vi "stripElementTags.vi"(8 "error in (no error)":errorcluster, 10 "XMLContents In":string, 11 "ReadElement in":refnum<class "XMLParser.lvclass">) -> (0 "error out":errorcluster, 1 "Contents":string, 2 "ParentTag":string, 3 "ReadElement out":refnum<class "XMLParser.lvclass">)   [LabVIEW 2014, in "XML.lvlib" / "XMLParser.lvclass"]
doc: "This method checks the open and close tags, and returns whatever is in the middle. This will not work if there are attributes in the parent tag."
uses:
  <userlib>/Common/XML/XMLParser/XMLParser.lvclass
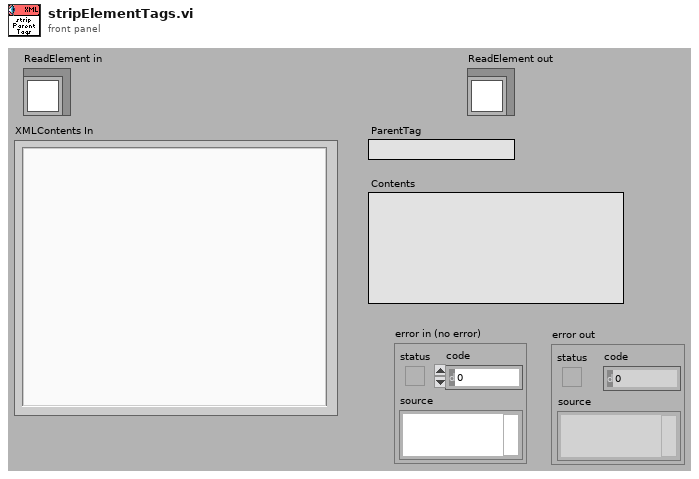
[diagram p1: front panel]
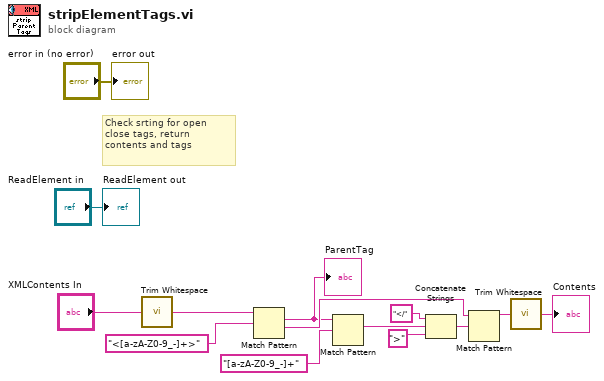
[diagram p0: block diagram]
diagram:
  # "Check srting for open close tags, return contents and tags"
  n1 = call <vilib>:"Trim Whitespace.vi"("string"="XMLContents In") -> ("trimmed string"=w11:string)  [unwired: 1 in]
  n2 = Match Pattern(string=w11, regular expression="<[a-zA-Z0-9_-]+>") -> (match substring=w5:string, after substring=w10:string)  [unwired: 1 in, 2 out]
  "ParentTag" <- w5
  n3 = Match Pattern(string=w5, regular expression="[a-zA-Z0-9_-]+") -> (match substring=w7:string)  [unwired: 1 in, 3 out]
  n4 = Concatenate Strings("</" ("string"), w7, ">" ("string")) -> (w8:string)
  n5 = Match Pattern(string=w10, regular expression=w8) -> (before substring=w12:string)  [unwired: 1 in, 3 out]
  n6 = call <vilib>:"Trim Whitespace.vi"("string"=w12) -> ("trimmed string"=→"Contents":string)  [unwired: 1 in]
  "error out" <- "error in (no error)"
  "ReadElement out" <- "ReadElement in"
